vi "gentec-SOLO-PE.set Trigger Level.vi"(8 "error in (no error)":errorcluster, 10 "Trigger Level (2%)":u32=2, 11 "VISA Refnum in":refnum<visa-resource-name>) -> (0 "error out":errorcluster, 1 "Acknoledged?":bool, 2 "Error":string, 3 "VISA Refnum out":refnum<visa-resource-name>, 4 "Timeout":bool)   [LabVIEW 2014, in "gentec-SOLO-PE - Driver.lvlib"]
doc: "Serts the Trigger Level in Percent."
uses:
  gentec-SOLO-PE - Driver.lvlib
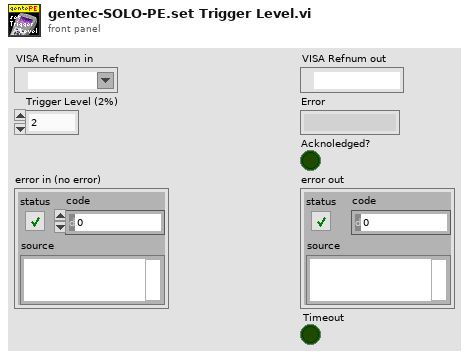
[diagram p1: front panel]
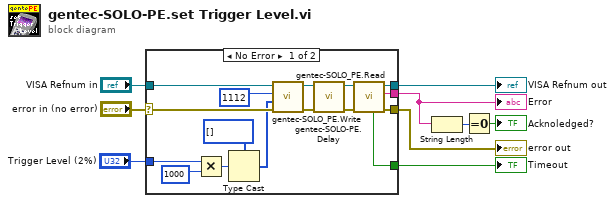
[diagram p0: block diagram]
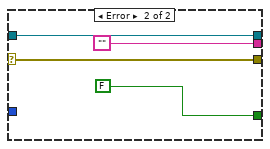
[diagram p2: hidden frame]
diagram:
  n1 = case shown="No Error" "error in (no error)" {
    selector: "error in (no error)" -> [w17 w28]
    tunnel: [w15 w28] -> w9
    tunnel: [w25 w29] -> w8
    tunnel: [w16 ""] -> w3
    tunnel: [w24 FALSE ("Timeout")] -> w7
    tunnel: "VISA Refnum in" -> [w19 w29]
    tunnel: "Trigger Level (2%)" -> [w12 _]
    frame No Error {
      n2 = Multiply(x=w12, y=u32 1000) -> (x*y=w11:u32)
      n3 = Type Cast(type=u32[] [], x=w11) -> (*(type *) &x=w13:u32[])
      n4 = call "gentec-SOLO_PE.Write.vi"("error in (no error)"=w17, "Parameters (Empty)"=w13, "Command Handle"=u16 1112, "VISA Refnum in"=w19) -> ("error out"=w22:errorcluster, "VISA Refnum out"=w20:refnum<visa-resource-name>)  [unwired: 6 in]
      n5 = call "gentec-SOLO-PE.Delay.vi"("error in (no error)"=w22, "VISA resource In"=w20) -> ("error out"=w23:errorcluster, "VISA resource Out"=w21:refnum<visa-resource-name>)  [unwired: 4 in]
      n6 = call "gentec-SOLO_PE.Read.vi"("error in (no error)"=w23, "VISA Refnum in"=w21) -> ("error out"=w15:errorcluster, "Error"=w16:string, "VISA Refnum out"=w25:refnum<visa-resource-name>, "Timeout"=w24:bool)  [unwired: 5 in, 1 out]
    }
    frame Error {
    }
  }
  "error out" <- w9
  "VISA Refnum out" <- w8
  "Error" <- w3
  "Timeout" <- w7
  n7 = String Length(string=w3) -> (length=w2:i32)
  n8 = Equal To 0?(x=w2) -> (x = 0?=→"Acknoledged?":bool)
